vi "Ivan_method.vi"() -> ()   [LabVIEW 2017]
uses:
  ONNX Class/ONNX Class.lvclass
  <vilib>/Utility/file.llb/Read Delimited Spreadsheet (DBL).vi
panel:
  out "time":u32
  out "Variant out":variant
  out "Y predicted":sgl
  out "X predicted":sgl
  out "Reshaped input":dbl[](array[numeric])
  out "X and Y std":sgl[][](array[numeric])
  out "initialized array 2":sgl[][](array[numeric])
  out "X and Y means":sgl[][](array[numeric])
  out "initialized array":sgl[][](array[numeric])
  out "raw data":dbl[][](array[numeric])
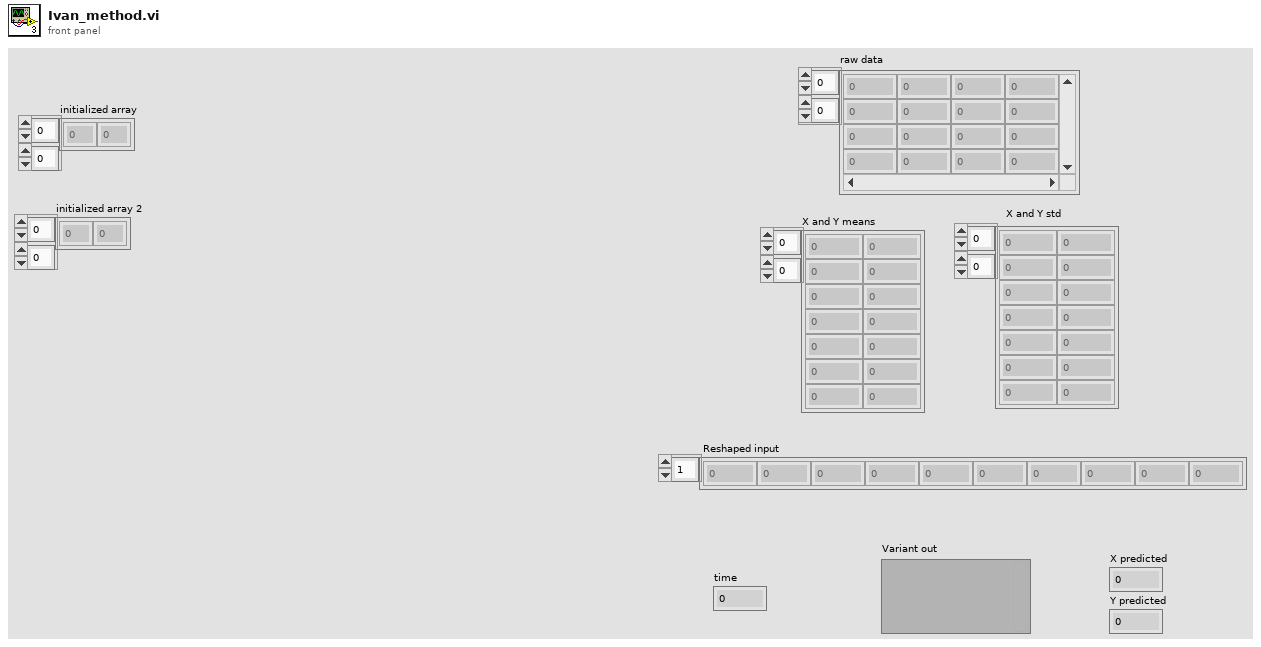
[diagram p1: front panel]
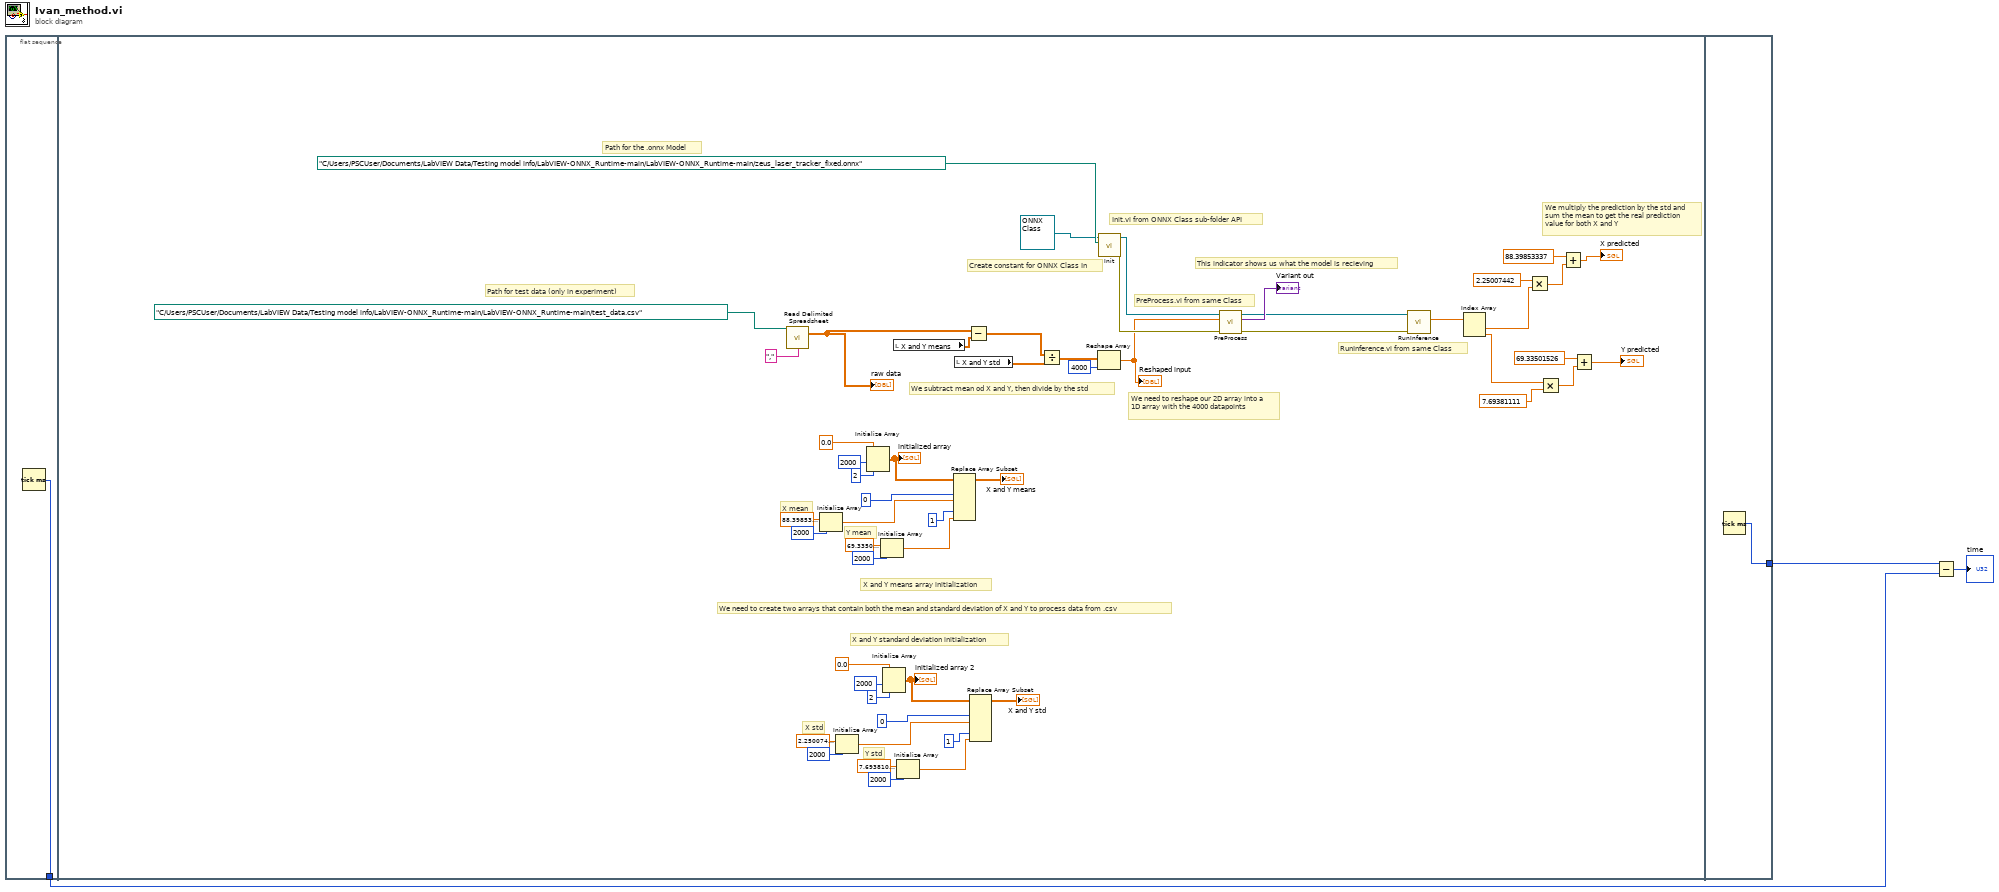
[diagram p0: block diagram]
diagram:
  n1 = flat-sequence {
    tunnel: [w4] -> w2
    tunnel: [w58] -> w3
    frame #0 {
      n2 = Tick Count (ms)() -> (millisecond timer value=w4:u32)
    }
    frame #1 {
      # "We multiply the prediction by the std and sum the mean to get the real prediction value for both X and Y"
      # "This indicator shows us what the model is recieving"
      # "RunInference.vi from same Class"
      # "PreProcess.vi from same Class"
      # "Init.vi from ONNX Class sub-folder API"
      # "Create constant for ONNX Class In"
      # "We need to reshape our 2D array into a 1D array with the 4000 datapoints"
      # "We subtract mean od X and Y, then divide by the std"
      # "Y std"
      # "X std"
      # "Y mean"
      # "X mean"
      # "We need to create two arrays that contain both the mean and standard deviation of X and Y to process data from .csv"
      # "Path for test data (only in experiment)"
      # "Path for the .onnx Model"
      # "X and Y standard deviation initialization"
      # "X and Y means array initialization"
      n3 = call-poly <vilib>:"Read Delimited Spreadsheet.vi"("file path (dialog if empty)"=path "C:/Users/PSCUser/Documents/LabVIEW Data/Testing model info/LabVIEW-ONNX_Runtime-main/LabVIEW-ONNX_Runtime-main/test_data.csv", "delimiter (\\t)"="," ("delimiter (\\t)")) -> ("all rows"=w42:dbl[][])  [unwired: 8 in, 5 out]
      "raw data" <- w42
      n4 = Initialize Array(sgl 88.39854 ("element"), 2000 ("dimension size")) -> (w46:sgl[])
      n5 = Initialize Array(sgl 2.2500744 ("element"), 2000 ("dimension size")) -> (w5:sgl[])
      n6 = Initialize Array(sgl 0.0 ("element"), 2000 ("dimension size"), 2 ("dimension size")) -> (w52:sgl[][])
      "initialized array" <- w52
      n7 = Initialize Array(sgl 69.335014 ("element"), 2000 ("dimension size")) -> (w43:sgl[])
      n8 = Initialize Array(sgl 0.0 ("element"), 2000 ("dimension size"), 2 ("dimension size")) -> (w36:sgl[][])
      "initialized array 2" <- w36
      n9 = local read "X and Y means"() -> (w41:sgl[][])
      n10 = Initialize Array(sgl 7.693811 ("element"), 2000 ("dimension size")) -> (w28:sgl[])
      n11 = Replace Array Subset(array=w52, new element #1=w46, index (col) #1=0 ("disabled index (col)"), new element #2=w43, index (col) #2=1 ("disabled index (col)")) -> (→"X and Y means":sgl[][])  [unwired: 2 in]
      n12 = local read "X and Y std"() -> (w27:sgl[][])
      n13 = Subtract(x=w42, y=w41) -> (x-y=w40:dbl[][])
      n14 = Replace Array Subset(array=w36, new element #1=w5, index (col) #1=0 ("disabled index (col)"), new element #2=w28, index (col) #2=1 ("disabled index (col)")) -> (→"X and Y std":sgl[][])  [unwired: 2 in]
      n15 = Divide(x=w40, y=w27) -> (x/y=w26:dbl[][])
      n16 = Reshape Array(w26, 4000 ("dimension size")) -> (w6:dbl[])
      "Reshaped input" <- w6
      n17 = call-dynamic "Init.vi"("ONNX Path"=path "C:/Users/PSCUser/Documents/LabVIEW Data/Testing model info/LabVIEW-ONNX_Runtime-main/LabVIEW-ONNX_Runtime-main/zeus_laser_tracker_fixed.onnx", "ONNX Class in"=refnum<class "ONNX Class.lvclass"> refnum) -> ("error out"=w7:errorcluster, "ONNX Class out"=w8:refnum<class "ONNX Class.lvclass">)  [unwired: 7 in, 1 out]
      n18 = call-dynamic "PreProcess.vi"("error in (no error)"=w7, "Variant in"=w6, "ONNX Class in"=w8) -> ("error out"=w10:errorcluster, "Variant out"=→"Variant out":variant, "ONNX Class out"=w9:refnum<class "ONNX Class.lvclass">)  [unwired: 6 in]
      n19 = call-dynamic "RunInference.vi"("error in (no error)"=w10, "ONNX Class in"=w9) -> ("Output Buffer"=w11:sgl[])  [unwired: 7 in, 2 out]
      n20 = Index Array(array=w11) -> (element #1=w15:sgl, element #2=w20:sgl)  [unwired: 2 in]
      n21 = Multiply(x=2.25007442, y=w15) -> (x*y=w14:dbl)
      n22 = Multiply(x=w20, y=7.69381111 ("x")) -> (x*y=w18:dbl)
      n23 = Add(x=88.39853337, y=w14) -> (x+y=→"X predicted":dbl)
      n24 = Add(x=69.33501526, y=w18) -> (x+y=→"Y predicted":dbl)
    }
    frame #2 {
      n25 = Tick Count (ms)() -> (millisecond timer value=w58:u32)
    }
  }
  n26 = Subtract(x=w3, y=w2) -> (x-y=→"time":u32)
